vi "Instrument Do Core.vi"(8 "error in (no error)":errorcluster, 9 "Instrument in":refnum<class "Instrument Driver.lvclass">, 10 "Actor in":refnum<class "Actor.lvclass">, 11 "DMM Msg in":refnum<class "DMM Msg.lvclass">) -> (0 "error out":errorcluster, 1 "Instrument out":refnum<class "Instrument Driver.lvclass">, 2 "Actor out":refnum<class "Actor.lvclass">, 3 "DMM Msg out":refnum<class "DMM Msg.lvclass">, 5 "Data":refnum<class "Data.lvclass">)   [LabVIEW 2020, in "DMM Msg.lvlib" / "DMM Msg.lvclass"]
doc: "Message interaction with any instrument is handled by the Instrument Do Core.\n\nThe default implementation does nothing."
uses:
  DMM Msg.lvclass
  PPL/HDH.Actor Framework.Core.Actor.lvlibp/1abvi3w/vi.lib/ActorFramework/Actor/Actor.lvclass
  PPL/HDH.Data.Generic.lvlibp/Data.lvclass
  PPL/HDH.Actor Framework.Core.Instrument Driver.lvlibp/Instrument Driver/Instrument Driver.lvclass
  PPL/HDH.Actor Framework.Core.Instrument Handler.lvlibp/Messages/Instrument Msg/Instrument Msg.lvclass
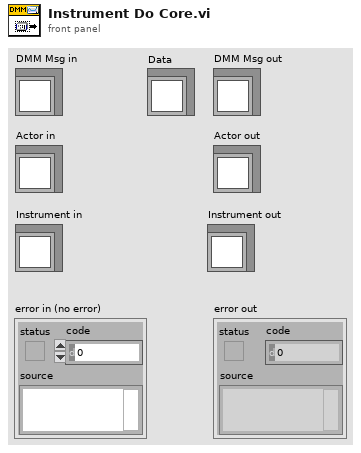
[diagram p1: front panel]
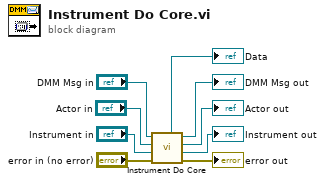
[diagram p0: block diagram]
diagram:
  n1 = call-parent "Instrument Do Core.vi"("error in (no error)"="error in (no error)", "Instrument in"="Instrument in", "Actor in"="Actor in", "Instrument Msg in"="DMM Msg in") -> ("error out"=→"error out":errorcluster, "Instrument out"=→"Instrument out":refnum<class "Instrument Driver.lvclass">, "Actor out"=→"Actor out":refnum<class "Actor.lvclass">, "Instrument Msg out"=→"DMM Msg out":refnum<class "DMM Msg.lvclass">, "Data"=→"Data":refnum<class "Data.lvclass">)  [unwired: 3 in]
